vi "SetControlValues.vi"(5 "Signaling (true)":bool=TRUE, 7 "application reference (local)":refnum<vi>, 8 "error in":errorcluster, 11 "ControlValueList":string) -> (0 "error out":errorcluster)   [LabVIEW 2019]
uses:
  <vilib>/regexp/Match Regular Expression.xnode
panel:
  # "VIName1\nControl1=Value1\nControl2=Value2\n\n// Comment\nVIName2\nControl1=Value1\nControl2=Value2"
  # "VI名に続いて\nコントロール名=値　の行を複数並べる\n\n異なる VI への書き込みは空行を挟んで続ける。\n// から始まる行はコメント\n行の途中から // でコメントを入れることはできない"
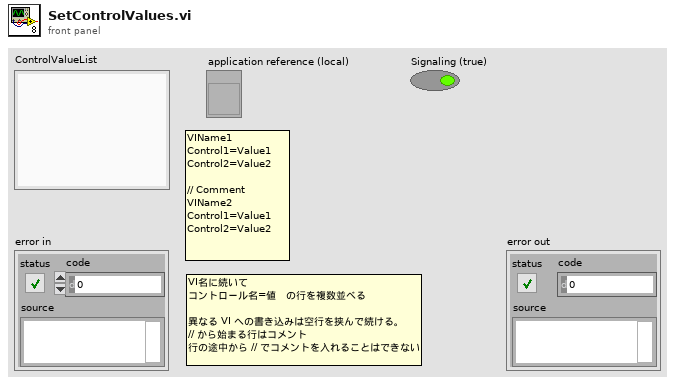
[diagram p1: front panel]
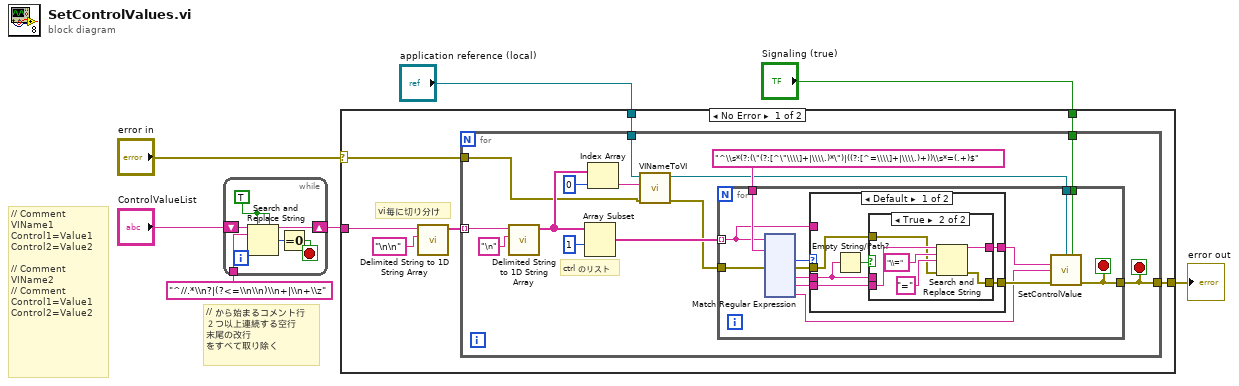
[diagram p0: block diagram]
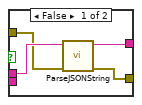
[diagram p2: hidden frame]
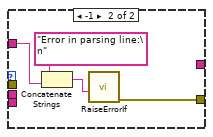
[diagram p3: hidden frame]
diagram:
  # "// から始まるコメント行\n２つ以上連続する空行\n末尾の改行\nをすべて取り除く"
  # "// Comment\nVIName1\nControl1=Value1\nControl2=Value2\n\n// Comment\nVIName2\n// Comment\nControl1=Value1\nControl2=Value2"
  n1 = while {
    shift-right: [w13] -> w3
    shift-left: "ControlValueList" -> [w11]
    tunnel: "^//.*\\n?|(?<=\\n\\n)\\n+|\\n+\\z" ("search string") -> [w8]
    stop <- w9 stop-if-true
    w12 = TRUE ("multiline? (F)")
    n2 = Search and Replace String(replace all?=w12, multiline?=w12, input string=w11, search string=w8) -> (result string=w13:string, number of replacements=w10:i32)  [unwired: 4 in, 2 out]
    n3 = Equal To 0?(x=w10) -> (x = 0?=w9:bool)
  }
  n4 = case shown="No Error" "error in" {
    selector: "error in" -> [w14 w189]
    tunnel: w3 -> [w19 _]
    tunnel: "Signaling (true)" -> [w17 _]
    tunnel: "application reference (local)" -> [w16 _]
    tunnel: [w15 w189] -> w5
    frame No Error {
      # "vi毎に切り分け"
      n5 = call <vilib>:"Delimited String to 1D String Array.vi"("delimiter"="\n\n", "delimited string"=w19) -> ("string array"=w18:string[])  [unwired: 9 in]
      n6 = for {
        tunnel: w18 -> [w30] mode=indexing
        tunnel: w17 -> [w27]
        tunnel: w16 -> [w26]
        tunnel: [w22] -> w15
        tunnel: w14 -> [w21]
        stop <- w22 stop-if-true
        # "ctrl のリスト"
        n7 = call <vilib>:"Delimited String to 1D String Array.vi"("delimiter"="\n", "delimited string"=w30) -> ("string array"=w34:string[])  [unwired: 9 in]
        n8 = Array Subset(array=w34, index=1) -> (w29:string[])  [unwired: 1 in]
        n9 = Index Array(array=w34, index=0) -> (element=w25:string)
        n10 = call "VINameToVI.vi"("error in (no error)"=w21, "vi"=w25, "Application in"=w26) -> ("error out"=w23:errorcluster, "VI out"=w24:refnum<vi>)  [unwired: 7 in]
        n11 = for {
          tunnel: w29 -> [w43] mode=indexing
          tunnel: "^\\s*(?:(\"(?:[^\"\\\\]+|\\\\.)*\")|((?:[^=\\\\]+|\\\\.)+))\\s*=(.+)$" -> [w47]
          tunnel: w27 -> [w39]
          tunnel: w24 -> [w38]
          tunnel: w23 -> [w37]
          tunnel: [w35] -> w22
          stop <- w35 stop-if-true
          n12 = xnode "Match Regular Expression"("input string"=w43, "regular expression"=w47, "error in"=w37) -> ("offset past match"=w46:i32, "error out"=w36:errorcluster, "submatch 1"=w45:string, "submatch 2"=w44:string, "submatch 3"=w40:string)  [unwired: 3 in, 3 out]
          n13 = case shown="Default" w46 {
            tunnel: w45 -> [w52 _]
            tunnel: w44 -> [w51 _]
            tunnel: [w50 _] -> w41
            tunnel: w43 -> [_ w66]
            tunnel: [w48 w64] -> w42
            tunnel: w36 -> [w49 _]
            frame Default {
              n14 = Empty String/Path?(string/path=w52) -> (empty?=w53:bool)
              n15 = case shown="True" w53 {
                tunnel: w52 -> [w57 _]
                tunnel: w51 -> [_ w63]
                tunnel: [w56 w60] -> w50
                tunnel: w49 -> [w55 w59]
                tunnel: [w54 w58] -> w48
                frame False {
                  n16 = call "ParseJSONString.vi"("error in (no error)"=w55, "JSON string"=w57) -> ("error out"=w54:errorcluster, "string"=w56:string)  [unwired: 8 in]
                }
                frame True {
                  n17 = Search and Replace String(input string=w63, search string="\\=", replace string="=" ("replace string (\"\")"), error in=w59) -> (result string=w60:string, error out=w58:errorcluster)  [unwired: 4 in, 2 out]
                }
              }
            }
            frame -1 {
              n18 = Concatenate Strings("Error in parsing line:\n", w66) -> (w65:string)
              n19 = call "RaiseErrorIf.vi"("error message"=w65) -> ("error out"=w64:errorcluster)  [unwired: 10 in]
            }
          }
          n20 = call "SetControlValue.vi"("vi ref"=w38, "Signaling"=w39, "ctrl"=w41, "Value (JSON)"=w40, "error in (no error)"=w42) -> ("error out"=w35:errorcluster)  [unwired: 10 in]
        }
      }
    }
    frame Error {
    }
  }
  "error out" <- w5
